vi "SL TAGS Get Values.vi"(8 "error in (no error)":errorcluster, 9 "Tag Scope":T1=enum."Server", 10 "Tag Type":T2, 11 "EEISysLink in":refnum<class "EEISysLink.lvclass">) -> (0 "error out":errorcluster, 2 "Tag Values":T3[](array[typedef]), 3 "EEISysLink out":refnum<class "EEISysLink.lvclass">)   [LabVIEW 2017, in "EEISysLink.lvclass"]
doc: "Will return the current value of all selected tag types. Will retrieve the values within the selected scope as follows. \n\nServer = Get updated values from the SystemLink server, update the class tag values, and return them.\nLocal = Return the values of the class tags\n\nJames Tillett P.E.\nEndeavor Engineering Inc.\nwww.endeavoreng.com"
uses:
  EEISysLink.lvclass
  Controls/SL Tag Value.ctl
  Controls/SL Tag Data Type.ctl
  Controls/SL Tag Type.ctl
  Controls/SL Tag Scope.ctl
  EEISysLink.lvclass/EEISysLink.ctl
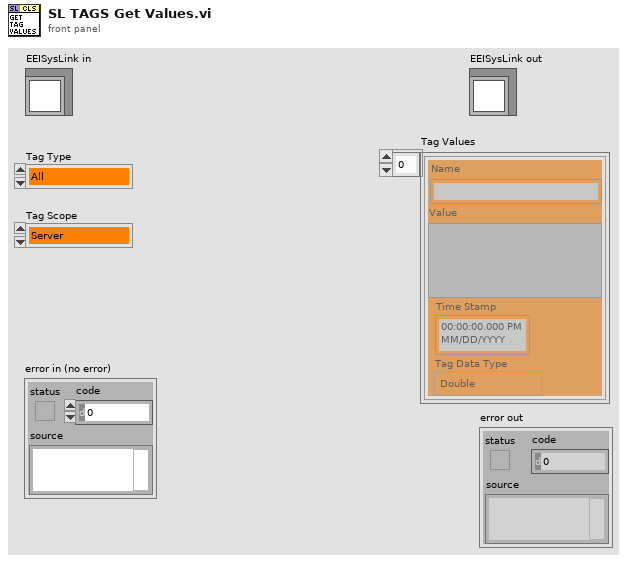
[diagram p1: front panel]
types:
  T1 = typedef "EEISysLink.lvclass/SL Tag Scope.ctl" = enum16{"Local", "Server"}
  T2 = typedef "EEISysLink.lvclass/SL Tag Type.ctl" = enum16{"All", "Supervisor", "Worker"}
  T3 = typedef "SL Tag Value.ctl" = cluster{"Value":variant, "Time Stamp":timestamp, "Tag Data Type":T4, "Name":string}
  T4 = typedef "EEISysLink.lvclass/SL Tag Data Type.ctl" = enum16{"Double", "Integer", "String", "Boolean", "Waveform"}
  T5 = typedef "EEISysLink.lvclass/SL Tag.ctl" = cluster{"Class Properties":T6, "SL Tag":refnum<class "NI Skyline Tag.lvclass">, "SystemLink Cluster":T9, "Class Value":variant}
  T6 = typedef "EEISysLink.lvclass/SL Tag Properties.ctl" = cluster{"Class Data Type":T4, "Name":string, "Description":string, "Interpolation Method":T7, "Unit of Measure":T8, "Maximum Interpolation":string, "Role":T2}
  T7 = typedef "EEISysLink.lvclass/SL Tag Interpolation Method.ctl" = enum16{"linear", "pilinear", "step"}
  T8 = typedef "EEISysLink.lvclass/SL Tag Unit of Measure.ctl" = enum16{"no units", "Second", "Hour", "Minute", "Day", "Year", "Month", "Week", "Foot", "Yard", "Meter", "Centimeter", "Inch", "Mile", "Nautical Mile", "Miles per Hour", "Meters per second", "Square meter", "Cubic meter", "Cubic centimeter", "Cubic inch", "Liter", "Gallon", "Gallons dry US", "Gallon UK", "Percent", "Revolutions per minute", "Revolution", "Degree angle", "Astronomical Unit", "Atom", "Atomic mass", "Bar", "Byte", "C (speed of light)", "Curie", "Decibel", "Electron Volt", "Ounce", "Knot", "G", "Grade", "Are", "Hectare", "Faraday", "Franklin", "Gilbert", "Erg", "Lambert", "Maxwell", "Gauss", "Electron mass", "Kilogram force", "Pound force", "Rad", "Centiradian", "Sphere", "Mach", "Fluid Ounces", "Fluid Ounces UK", "Fahrenheit", "Celsius", "Kelvin", "Rankine", "Gram", "Kilogram", "Pound", "Short/US Ton", "Long/UK ton", "Metric ton", "Mole", "Pounds per square inch", "Inches water column", "Torr", "Millitorr", "Millimeter mercury", "Inches mercury", "Bar (2)", "Atmosphere", "Pascal", "Watt", "kiloWatt", "Horsepower", "Kilowatt Hour", "British thermal units", "Millions of BTU", "Ampere", "Candela", "Radian", "Steradian", "Bit", "Hertz", "Newton", "Joule", "Coulomb", "Volt", "Farad", "Ohm", "Siemens", "Weber", "Tesla", "Henry", "Lumen", "Lux", "Becqueral", "Gray", "Sievert", "Katal", "Angstrom", "Light Year", "Parsec", "Point", "Pixel", "Dyne", "Kilogram force (2)", "Pound force (2)", "Rem", "Rutherford", "Roentgen"}
  T9 = typedef "NI Skyline Tag.lvlib/Tag Cluster.ctl" = cluster{"Path":string, "Data Type":T10, "Value":variant, "Time Stamp":timestamp}
  T10 = typedef "NI Skyline Tag.lvlib/DataType.ctl" = enum32{"Double", "Integer", "String"}
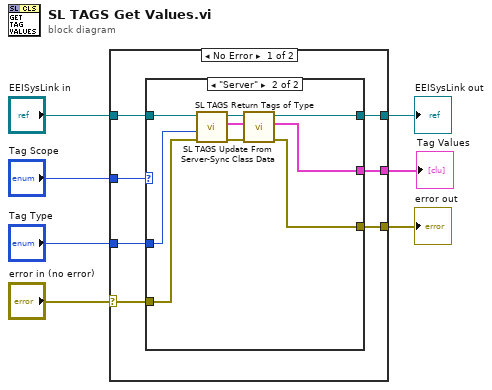
[diagram p0: block diagram]
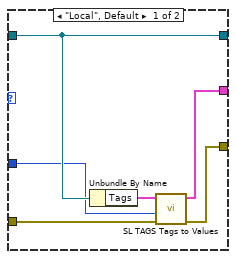
[diagram p2: hidden frame]
diagram:
  n1 = case shown="No Error" "error in (no error)" {
    selector: "error in (no error)" -> [w9 w31]
    tunnel: [w8 w31] -> w6
    tunnel: [w12 w30] -> w4
    tunnel: "EEISysLink in" -> [w13 w30]
    tunnel: "Tag Scope" -> [w14 _]
    tunnel: "Tag Type" -> [w11 _]
    tunnel: [w10 _] -> w1
    frame No Error {
      n2 = case shown="\"Server\"" w14 {
        tunnel: w13 -> [w20 w28]
        tunnel: [w20 w29] -> w12
        tunnel: w11 -> [w18 w27]
        tunnel: [w16 w22] -> w10
        tunnel: w9 -> [w17 w26]
        tunnel: [w15 w21] -> w8
        frame "Local", Default {
          n3 = Unbundle By Name(w20) -> ("Tags"=w19:T5[])
          n4 = call "SL TAGS Tags to Values.vi"("error in (no error)"=w17, "Tag Type"=w18, "Tags"=w19) -> ("error out"=w15:errorcluster, "Tag Values"=w16:T3[])  [unwired: 7 in]
        }
        frame "Server" {
          n5 = call "SL TAGS Return Tags of Type.vi"("error in (no error)"=w26, "Tag Type"=w27, "EEISysLink in"=w28) -> ("error out"=w23:errorcluster, "Tags of Type"=w25:T5[], "EEISysLink out"=w24:refnum<class "EEISysLink.lvclass">)  [unwired: 6 in]
          n6 = call "SL TAGS Update From Server-Sync Class Data.vi"("error in (no error)"=w23, "Tags to Update"=w25, "EEISysLink in"=w24) -> ("error out"=w21:errorcluster, "Updated Tag Values"=w22:T3[], "EEISysLink out"=w29:refnum<class "EEISysLink.lvclass">)  [unwired: 6 in]
        }
      }
    }
    frame Error {
    }
  }
  "error out" <- w6
  "EEISysLink out" <- w4
  "Tag Values" <- w1
